vi "INIT LED.vi"(8 "error in (no error)":errorcluster) -> (0 "error out":errorcluster)   [LabVIEW 2023]
uses:
  ctrl defs/ctrl LED init.ctl
  <vilib>/Rock Robotics/SystemInterfaces/DIO/FPGA_DIOPWMChannel.ctl
  ctrl defs/ctrl number of LEDs.ctl
  ctrl defs/ctrl LED PATTERNS.ctl
  Global INIT.vi
  <vilib>/Rock Robotics/WPI/MotorControl/WPI_MotorControlOpen SPARK.vi
  <vilib>/Rock Robotics/Network Tables/NT Write Number.vi
panel:
  out "LED init":T1={"PWM Channel"=enum."PWM 0", "refnum name"="LED", "#LEDS"=0, "initial output"=0.51, "stack name"="LED/value", "Installed?"=FALSE, "pattern"=0} {"pattern" items=["<<Select a pattern>>", "Rainbow, Rainbow palette", "Rainbow, Party palette", "Rainbow, Ocean palette", "Rainbow, Lava palette", "Rainbow, Forest palette", "Rainbow with glitter", "Confetti", "Shot, Red", "Shot, Blue", "Shot, White", "Sinelon, Rainbow palette", "Sinelon, Party palette", "Sinelon, Ocean palette", "Sinelon, Lava palette", "Sinelon, Forest palette", "BPM, Rainbow palette", "BPM, Party palette", "BPM, Ocean palette", "BPM, Lava palette", "BPM, Forest palette", "Fire, Medium", "Fire, Large", "Twinkles, Rainbow palette", "Twinkles, Party palette", "Twinkles, Ocean palette", "Twinkles, Lava palette", "Twinkles, Forest palette", "Color Waves, Rainbow palette", "Color Waves, Party palette", "Color Waves, Ocean palette", "Color Waves, Lava palette", "Color Waves, Forest palette", "Larson Scanner, Red", "Larson Scanner, Gray", "Light Chase, Red", "Light Chase, Blue", "Light Chase, Gray", "Heartbeat, Red", "Heartbeat, Blue", "Heartbeat, White", "Heartbeat, Gray", "Breath, Red", "Breath, Blue", "Breath, Gray", "Strobe, Red", "Strobe, Blue", "Strobe, Gold", "Strobe, White", "Color 1: End to End Blend to Black", "Color 1: Larson Scanner", "Color 1: Light Chase", "Color 1: Heartbeat Slow", "Color 1: Heartbeat Medium", "Color 1: Heartbeat Fast", "Color 1: Breath Slow", "Color 1: Breath Fast", "Color 1: Shot", "Color 1: Strobe", "Color 2: End to End Blend to Black", "Color 2: Larson Scanner", "Color 2: Light Chase", "Color 2: Heartbeat Slow", "Color 2: Heartbeat Medium", "Color 2: Heartbeat Fast", "Color 2: Breath Slow", "Color 2: Breath Fast", "Color 2: Shot", "Color 2: Strobe", "Color 1/2: Sparkle, 1 on 2", "Color 1/2: Sparkle 2 on 1", "Color 1/2: Gradient", "Color 1/2: BPM", "Color 1/2: End to End Blend 1 to 2", "Color 1/2: End to End Blend 2 to 1", "Color 1/2: setup pattern", "Color 1/2: Twinkles", "Color 1/2: Color Waves", "Color 1/2: Sinelon", "Solid Hot Pink", "Solid Dark Red", "Solid Red", "Solid Red Orange", "Solid Orange", "Solid Gold", "Solid Yellow", "Solid Lawn Green", "Solid Lime", "Solid Dark Green", "Solid Green", "Solid Blue Green", "Solid Aqua", "Solid Sky Blue", "Solid Dark Blue", "Solid Blue", "Solid Blue Violet", "Solid Violet", "Solid White", "Solid Gray", "Solid Dark Gray", "Solid Black"]}
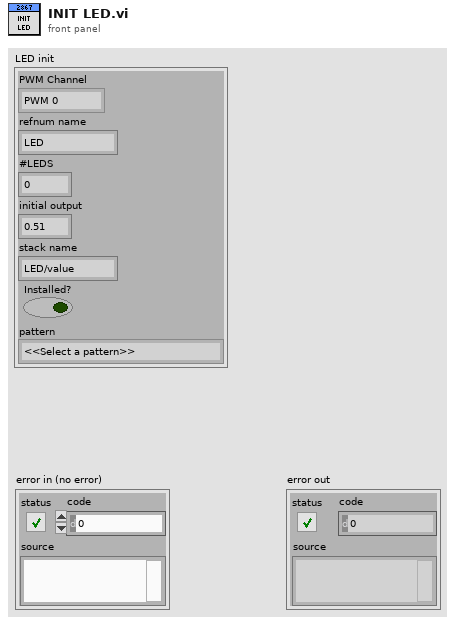
[diagram p1: front panel]
types:
  T1 = typedef "ctrl LED init.ctl" = cluster{"PWM Channel":T2, "refnum name":string, "#LEDS":T3, "initial output":dbl, "stack name":string, "Installed?":bool, "pattern":T4}
  T2 = typedef "FPGA_DIOPWMChannel.ctl" = enum8{"PWM 0", "PWM 1", "PWM 2", "PWM 3", "PWM 4", "PWM 5", "PWM 6", "PWM 7", "PWM 8", "PWM 9", "PWM MXP 0", "PWM MXP 1", "PWM MXP 2", "PWM MXP 3", "PWM MXP 4", "PWM MXP 5", "PWM MXP 6", "PWM MXP 7", "PWM MXP 8", "PWM MXP 9", "Invalid"}
  T3 = typedef "ctrl number of LEDs.ctl" = u16
  T4 = typedef "ctrl LED PATTERNS.ctl" = u16
  T5 = typedef "WPI_MotorControlDeviceRef.ctl" = cluster{"DeviceStatus":errorcluster, "Type":T6, "PWM":cluster{"PWM Channel":T2, "DeadBand":T7}, "CAN":cluster{"Device Number":u8, "SetOutput VI Ref":variant, "GetOutput VI Ref":variant, "Enable VI Ref":variant, "Disable VI Ref":variant, "Data":variant}, "Invert":bool, "DIO PWM":cluster{"PWM \"Enable\" Channel":T2, "DIOChannel":T8, "PWM Rate":dbl}}
  T6 = typedef "WPI_MotorControlType.ctl" = enum16{"PWM", "CAN", "DIO PWM"}
  T7 = typedef "WPI_PWMDeadband.ctl" = cluster{"Name":string, "maxPositivePwm":i32, "minPositivePwm":i32, "centerPwm":i32, "maxNegativePwm":i32, "minNegativePwm":i32, "angularRange":u16}
  T8 = typedef "FPGA_DIOChannel.ctl" = enum8{"DIO 0", "DIO 1", "DIO 2", "DIO 3", "DIO 4", "DIO 5", "DIO 6", "DIO 7", "DIO 8", "DIO 9", "DIO MXP 0", "DIO MXP 1", "DIO MXP 2", "DIO MXP 3", "DIO MXP 4", "DIO MXP 5", "DIO MXP 6", "DIO MXP 7", "DIO MXP 8", "DIO MXP 9", "DIO MXP 10", "DIO MXP 11", "DIO MXP 12", "DIO MXP 13", "DIO MXP 14", "DIO MXP 15", "SPI Port CS1", "SPI Port CS2", "SPI Port CS3", "SPI Port MISO", "SPI Port MOSI", "Invalid"}
  T9 = typedef "WPI_PWMDeviceRef.ctl" = cluster{"DeviceStatus":errorcluster, "PWM Channel":T2}
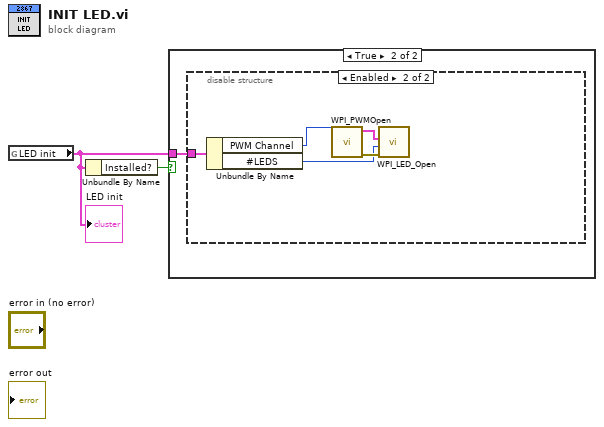
[diagram p0: block diagram]
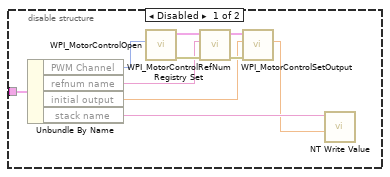
[diagram p3: hidden frame]
diagram:
  n1 = global read "Global INIT.vi" "LED init"() -> (w1:T1)
  "LED init" <- w1
  n2 = Unbundle By Name(w1) -> ("Installed?"=w2:bool)
  n3 = case shown="True" w2 {
    tunnel: w1 -> [_ w3]
    frame False {
    }
    frame True {
      n4 = disable-structure shown="Enabled" {
        disable-tunnel: w3 -> [w9 w16]
        frame Disabled {
          n5 = Unbundle By Name(w9) -> ("PWM Channel"=w8:T2, "refnum name"=w7:string, "initial output"=w6:dbl, "stack name"=w5:string)
          n6 = call-poly <vilib>:"WPI_MotorControlOpen.vi"("PWM Channel"=w8) -> ("error out"=w13:errorcluster, "MotorControlDeviceRef"=w12:T5)  [unwired: 9 in]
          n7 = call <vilib>:"WPI_MotorControlRefNum Registry Set.vi"("error in (no error)"=w13, "refnum name"=w7, "MotorControlDevRef"=w12) -> ("error out"=w11:errorcluster, "MotorControlDevRef"=w10:T5)  [unwired: 7 in]
          n8 = call <vilib>:"WPI_MotorControlSetOutput.vi"("error in (no error)"=w11, "Output"=w6, "MotorControlDevRef"=w10) -> ("Motor Output"=w4:dbl)  [unwired: 6 in, 2 out]
          n9 = call-poly <vilib>:"NT Write Value.vi"("value"=w4, "name"=w5) -> ()  [unwired: 9 in, 1 out]
        }
        frame Enabled {
          n10 = Unbundle By Name(w16) -> ("PWM Channel"=w14:T2, "#LEDS"=w15:T3)
          n11 = call <vilib>:"WPI_PWMOpen.vi"("PWM Channel"=w14) -> ("error out"=w17:errorcluster, "PWMDeviceRef"=w18:T9)  [unwired: 9 in]
          n12 = call <vilib>:"WPI_LED_Open.vi"("error in"=w17, "String Length"=w15, "PWMDeviceRef"=w18) -> ()  [unwired: 8 in, 1 out]
        }
      }
    }
  }
